vi "AB_API Build.vi"(8 "error in (no error)":errorcluster, 9 "collect dependencies?":bool, 10 "preview":bool, 11 "Build in":refnum<class "AB_Build.lvclass">) -> (0 "error out":errorcluster, 1 "Dependencies":T1[](array[typedef]), 2 "GeneratedFiles":path[](array[path]), 3 "Build out":refnum<class "AB_Build.lvclass">)   [LabVIEW 2020]
uses:
  <vilib>/AppBuilder/AB_Classes/Build/AB_Build.lvclass
  <vilib>/AppBuilder/AB_Dependency.ctl
  <vilib>/Utility/lvfile.llb/LVFileType.ctl
  <vilib>/Utility/lvfile.llb/NI_FileType.lvlib
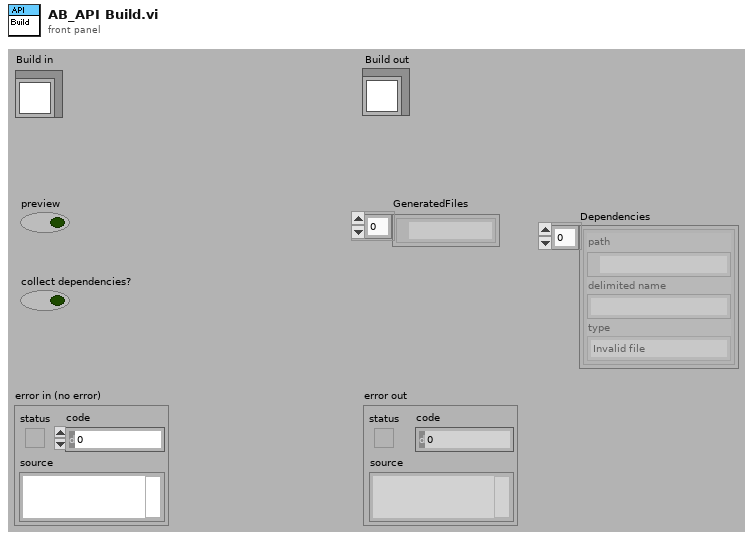
[diagram p1: front panel]
types:
  T1 = typedef "AB_Dependency.ctl" = cluster{"path":path, "delimited name":string, "type":T2}
  T2 = typedef "NI_FileType.lvlib/LVFileType.ctl" = enum32{"Invalid file", "Unknown type", "Instrument", "Control", "Polymorphic VI", "Project", "Library", "LVClass", "XControl", "XNode", "Shared library", ".NET assembly", "ActiveX interface", "CIN", "Run-time menu", "Palette menu", "Help file", "LLB", "XNode Edit Dependency", "Class Private Data Control", "Statechart", "MathScript .m file", "Ladder Diagram", "LVLibp", "XNode Build Dependency"}
  T3 = typedef "AB_Build.ctl" = cluster{"buildSpecName":string, "buildSpecDescription":string, "destinations":refnum<class "AB_Destination.lvclass">[], "exclusionOption":T4, "defaultLanguage":string, "supportedLanguages":string[], "excludedDirectories":path[], "buildContext":refnum<vi>, "buildObject":T5, "preview":bool, "programatic":bool, "progressBarEvents":T6, "userLog_Path":path, "preActionID":string, "preAction_Path":path, "postActionID":string, "postAction_Path":path, "eng_checkForBrokenVIs?":bool, "eng_verboseLinkerErrors?":bool, "localDest_Path":path, "targetDest_Path":path, "removeVIObject":u16, "cache":refnum<class "PreviewCache.lvclass">, "use cache":bool, "previewCache_ID":string, "buildCache_ID":string, "eng_TempLocalDest_Path":path, "eng_collectDependencies?":bool, "versionInfo":cluster{"buildVersion":cluster{"major":u16, "minor":u16, "patch":u16, "build":u16}, "autoIncrement":bool}, "eng_enableVIChecksums":bool}
  T4 = typedef "AB_Exclusion_Option.ctl" = cluster{"typedefs":bool, "polymorphicVIs":bool, "unusedLibraryItems":bool, "modifyLibraryFile":bool, "edit-timeDependencies":bool, "inlineVIs":bool, "dependent PPLs":bool, "dependent DLLs":bool}
  T5 = typedef "ItemRef.ctl" = u64
  T6 = typedef "provcom_ProgressBar_Events.ctl" = cluster{"newJob":refnum<user-event>, "newItem":refnum<user-event>, "errorMsg":T7, "cancel":refnum<user-event>}
  T7 = typedef "mxLvBuildError.ctl" = refnum<user-event>
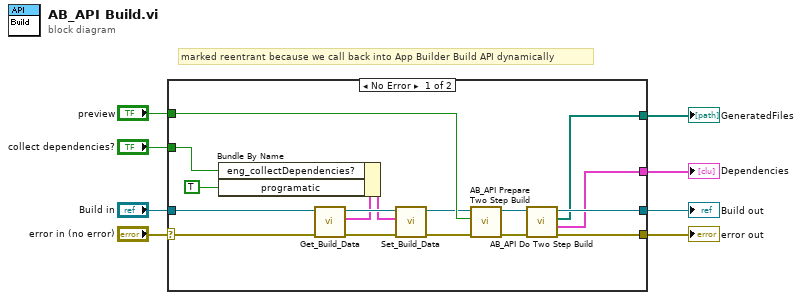
[diagram p0: block diagram]
diagram:
  # "marked reentrant because we call back into App Builder Build API dynamically"
  n1 = case shown="No Error" "error in (no error)" {
    selector: "error in (no error)" -> [w18 w27]
    tunnel: [w24 w27] -> w7
    tunnel: [w25 w26] -> w6
    tunnel: "Build in" -> [w17 w26]
    tunnel: [w23 _] -> w4
    tunnel: "preview" -> [w22 _]
    tunnel: [w10 _] -> w2
    tunnel: "collect dependencies?" -> [w9 _]
    frame No Error {
      n2 = call <vilib>:"Get_Build_Data.vi"("error in (no error)"=w18, "Class in"=w17) -> ("error out"=w12:errorcluster, "data"=w14:T3, "Class out"=w15:refnum<class "AB_Build.lvclass">)  [unwired: 7 in]
      n3 = Bundle By Name(cluster=w14, "eng_collectDependencies?"=w9, "programatic"=TRUE) -> (w13:T3)
      n4 = call <vilib>:"Set_Build_Data.vi"("error in (no error)"=w12, "data"=w13, "Class in"=w15) -> ("error out"=w19:errorcluster, "Class out"=w16:refnum<class "AB_Build.lvclass">)  [unwired: 7 in]
      n5 = call <vilib>:"AB_API Prepare Two Step Build.vi"("error in (no error)"=w19, "preview"=w22, "Build in"=w16) -> ("error out"=w20:errorcluster, "Class out"=w21:refnum<class "AB_Build.lvclass">)  [unwired: 6 in, 1 out]
      n6 = call <vilib>:"AB_API Do Two Step Build.vi"("error in (no error)"=w20, "Build in"=w21) -> ("error out"=w24:errorcluster, "Dependencies"=w10:T1[], "GeneratedFiles"=w23:path[], "Build out"=w25:refnum<class "AB_Build.lvclass">)  [unwired: 6 in]
    }
    frame Error {
    }
  }
  "error out" <- w7
  "Build out" <- w6
  "GeneratedFiles" <- w4
  "Dependencies" <- w2
